vi "Unloading_Status_Check_Unloaded.vi"() -> (3 "FEED CMPLT?":bool)   [LabVIEW 2017]
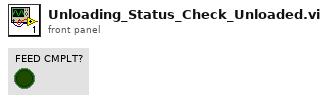
[diagram p1: front panel]
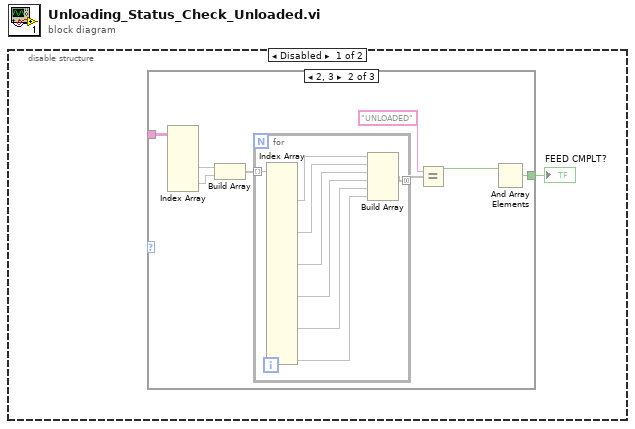
[diagram p0: block diagram]
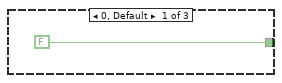
[diagram p2: hidden frame]
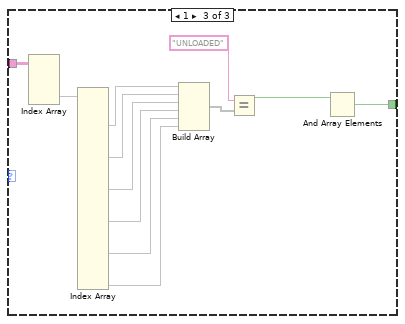
[diagram p3: hidden frame]
diagram:
  n1 = disable-structure shown="Disabled" {
    frame Disabled {
      n2 = case shown="2, 3" {
        selector: _ -> [_ _ _]
        tunnel: [_ w11 w31] -> w2
        tunnel: [FALSE w6 w22] -> w1
        frame 0, Default {
        }
        frame 2, 3 {
          n3 = Index Array(array=w11) -> (element #2=w10, element #3=w9)  [unwired: 6 in, 1 out]
          n4 = Build Array(w10, w9) -> (w8:void[])
          n5 = for {
            tunnel: w8 -> [w19] mode=indexing
            tunnel: [w12] -> w5 mode=concatenating
            n6 = Index Array(array=w19) -> (element #3=w18, element #7=w17, element #11=w16, element #15=w15, element #19=w14, element #23=w13)  [unwired: 23 in, 17 out]
            n7 = Build Array(w18, w17, w16, w15, w14, w13) -> (w12:void[])
          }
          n8 = Equal?(x="UNLOADED", y=w5) -> (x = y?=w4:bool)
          n9 = And Array Elements(Boolean array=w4) -> (logical AND=w6:bool)
        }
        frame 1 {
          n10 = Index Array(array=w31) -> (element #2=w30)  [unwired: 4 in, 1 out]
          n11 = Index Array(array=w30) -> (element #3=w28, element #7=w27, element #11=w26, element #15=w25, element #19=w24, element #23=w23)  [unwired: 23 in, 17 out]
          n12 = Build Array(w28, w27, w26, w25, w24, w23) -> (w21:void[])
          n13 = Equal?(x="UNLOADED", y=w21) -> (x = y?=w20:bool)
          n14 = And Array Elements(Boolean array=w20) -> (logical AND=w22:bool)
        }
      }
      "FEED CMPLT?" <- w1
    }
    frame Enabled {
    }
  }
